vi "Drive Distance Encoder.vi"(0 "Distance (in)":dbl=108.0, 1 "Gyro setpoint":dbl format="%.2f", 5 "Speed":dbl=0.8, 7 "Gyro gains":T1={"proportional gain (Kc)"=-0.08, "integral time (Ti, min)"=0.0, "derivative time (Td, min)"=0.0} {"derivative time (Td, min)" format="%.3f"; "integral time (Ti, min)" format="%.3f"; "proportional gain (Kc)" format="%.3f"}, 9 "Auto Notifiers In":T2, 11 "error in":errorcluster, 12 "Gyro Sync?":bool=TRUE) -> (10 "Auto Notifiers Out":T2, 15 "error out":errorcluster)   [LabVIEW 2014]
doc: "This VI will drive the specified distance at a specified motor output, it will not finish execution until it has reached its destination. The Gyro sync option (True by default) will sync the rotation to the read passed into the vi. Note this is a distance not a displacement (give us a positive)"
uses:
  Auto Notifiers.ctl
  Main/Arms/Arm clapper state.ctl
  Main/Arms/Arm State.ctl
  Utilities/Refname.ctl
  Utilities/Sensor Refname.ctl
  Utilities/RefnameToString.vi
  <vilib>/Rock Robotics/WPI/RobotDrive/WPI_RobotDriveGetSetRefNum.vi
  Utilities/Sensor Refname to String.vi
  <vilib>/addons/control/pid/pid.llb/PID (DBL).vi
  <vilib>/Rock Robotics/WPI/RobotDrive/WPI_RobotDriveArcadeDrive_Standard(NoSaturation).vi
  <vilib>/addons/control/pid/NI_PID_pid.lvlib
panel:
  in  "Max correction rate":dbl=1.0
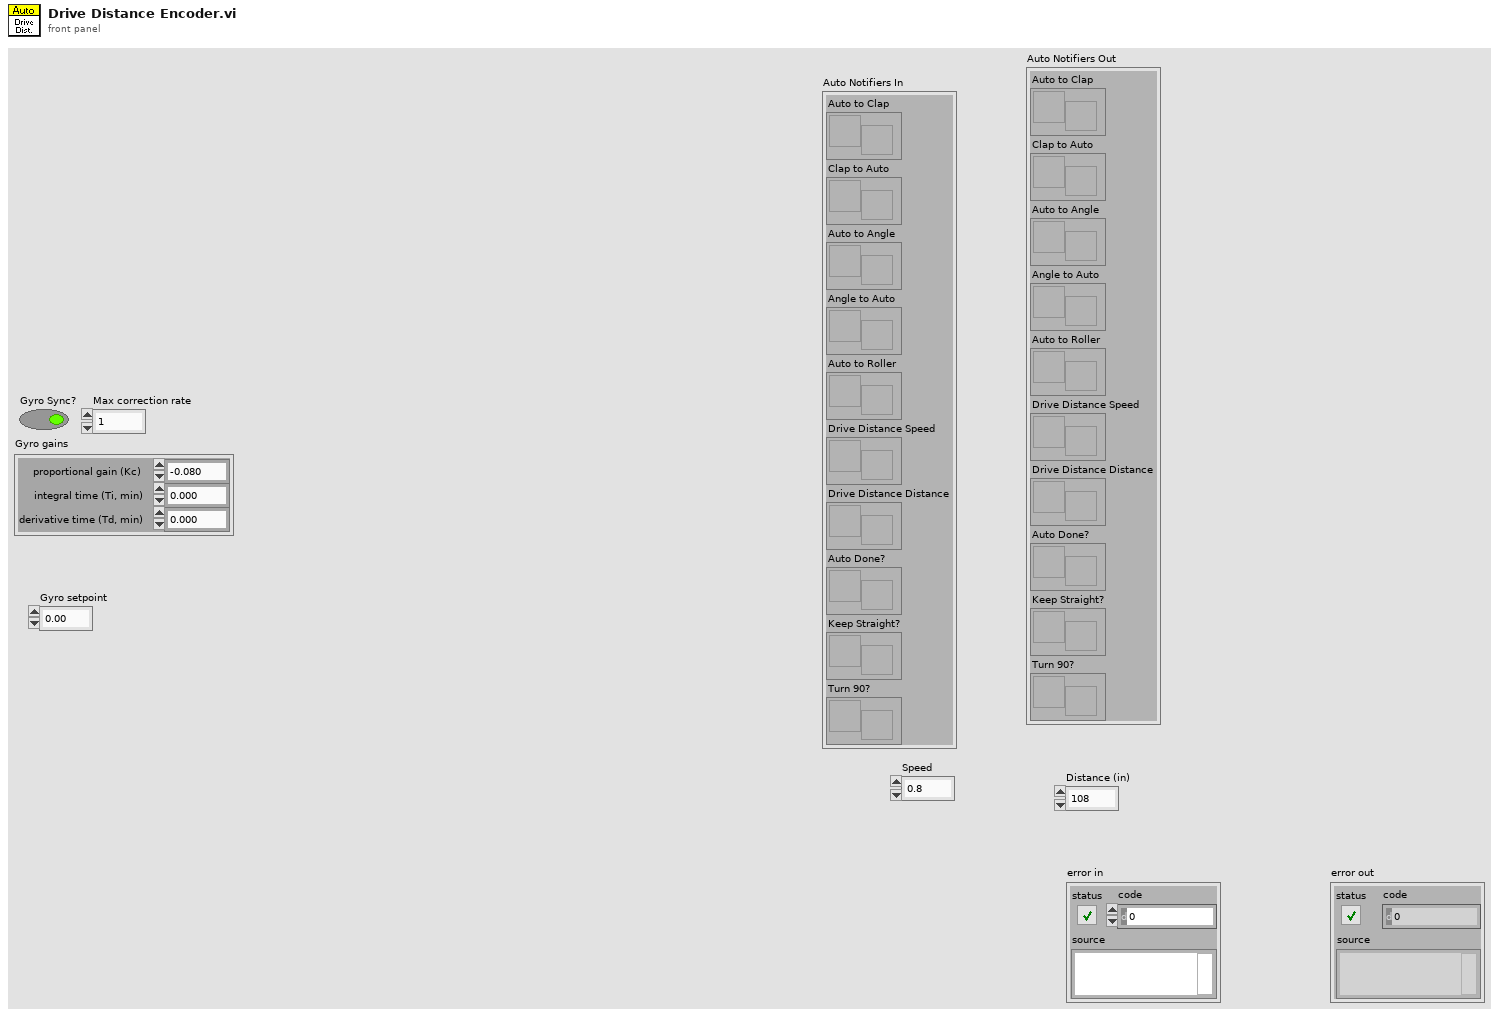
[diagram p1: front panel]
types:
  T1 = cluster{"proportional gain (Kc)":dbl, "integral time (Ti, min)":dbl, "derivative time (Td, min)":dbl}
  T2 = typedef "Auto Notifiers.ctl" = cluster{"Auto to Clap":refnum<notifier>, "Clap to Auto":refnum<notifier>, "Auto to Angle":refnum<notifier>, "Angle to Auto":refnum<notifier>, "Auto to Roller":refnum<notifier>, "Drive Distance Speed":refnum<notifier>, "Drive Distance Distance":refnum<notifier>, "Auto Done?":refnum<notifier>, "Keep Straight?":refnum<notifier>, "Turn 90?":refnum<notifier>}
  T3 = typedef "Refname.ctl" = enum16{"Gamepad 1", "Gamepad 2", "Drive Motors", "Strafe Motor", "Arm Clapper Motor", "Arm Angle", "Arm Belt Left", "Arm Belt Right", "Elevator 1", "Elevator 2", "Wiper"}
  T4 = typedef "WPI_RobotDriveDevRef.ctl" = cluster{"DevStatus":errorcluster, "Motors[]":T5[], "Square Inputs":bool, "Max Output":dbl}
  T5 = typedef "WPI_MotorControlDeviceRef.ctl" = cluster{"DeviceStatus":errorcluster, "Type":T6, "PWM":cluster{"Controller":T7, "PWM Channel":T8, "DeadBand":T9}, "CAN":cluster{"Device Number":u8, "Control Mode":T10, "Semaphore":T11, "Max Vout":dbl, "TalonSRX Control Mode":T12}, "Invert":bool, "TransformRef":T13, "InvTransformRef":T13}
  T6 = typedef "WPI_MotorControlType.ctl" = enum16{"PWM", "CAN", "CANTalonSRX"}
  T7 = typedef "FPGA_TypedefDigitalModule.ctl" = enum16{"Controller 1"}
  T8 = typedef "FPGA_DIOPWMChannel.ctl" = enum8{"PWM 0", "PWM 1", "PWM 2", "PWM 3", "PWM 4", "PWM 5", "PWM 6", "PWM 7", "PWM 8", "PWM 9", "PWM MXP 0", "PWM MXP 1", "PWM MXP 2", "PWM MXP 3", "PWM MXP 4", "PWM MXP 5", "PWM MXP 6", "PWM MXP 7", "PWM MXP 8", "PWM MXP 9", "Invalid"}
  T9 = typedef "WPI_PWMDeadband.ctl" = cluster{"Name":string, "maxPositivePwm":i32, "minPositivePwm":i32, "centerPwm":i32, "maxNegativePwm":i32, "minNegativePwm":i32, "angularRange":u16}
  T10 = typedef "WPI_CANJaguar_ControlMode.ctl" = enum8{"Percent VBus", "Current", "Speed", "Position", "Voltage"}
  T11 = typedef "Semaphore RefNum" = refnum<k1>
  T12 = typedef "WPI_CANTalonSRX_APIControlMode.ctl" = enum8{"Percent VBus", "Speed", "Position", "Slave", "Unchanged / Invalid"}
  T13 = typedef "WPI_PWMTransform_ConPane.ctl" = refnum<vi>
  T14 = typedef "Sensor Refname.ctl" = enum16{"Gyro", "Elevator Top LS", "Elevator Bottom LS", "Claw Outside LS", "Left Drive Encoder", "Right Drive Encoder", "Strafe Encoder", "Elevator Encoder", "Ultrasonic Forward", "Ultrasonic Back", "Arm Angle POT", "Arm Clapper POT", "Accelerometer", "Tote LS", "DIP 1", "DIP 2", "DIP 3", "DIP 4"}
  T15 = typedef "WPI_GyroDevRef.ctl" = cluster{"DevStatus":errorcluster, "Analog Module":T16, "Analog Channel":T17, "Offset":dbl, "Gain (VoltsPerDegree/Second)":dbl}
  T16 = typedef "FPGA_TypedefAnalogModule.ctl" = enum16{"Controller 1"}
  T17 = typedef "FPGA_AIChannel.ctl" = enum8{"AI 0", "AI 1", "AI 2", "AI 3", "AI MXP 0", "AI MXP 1", "AI MXP 2", "AI MXP 3", "Invalid"}
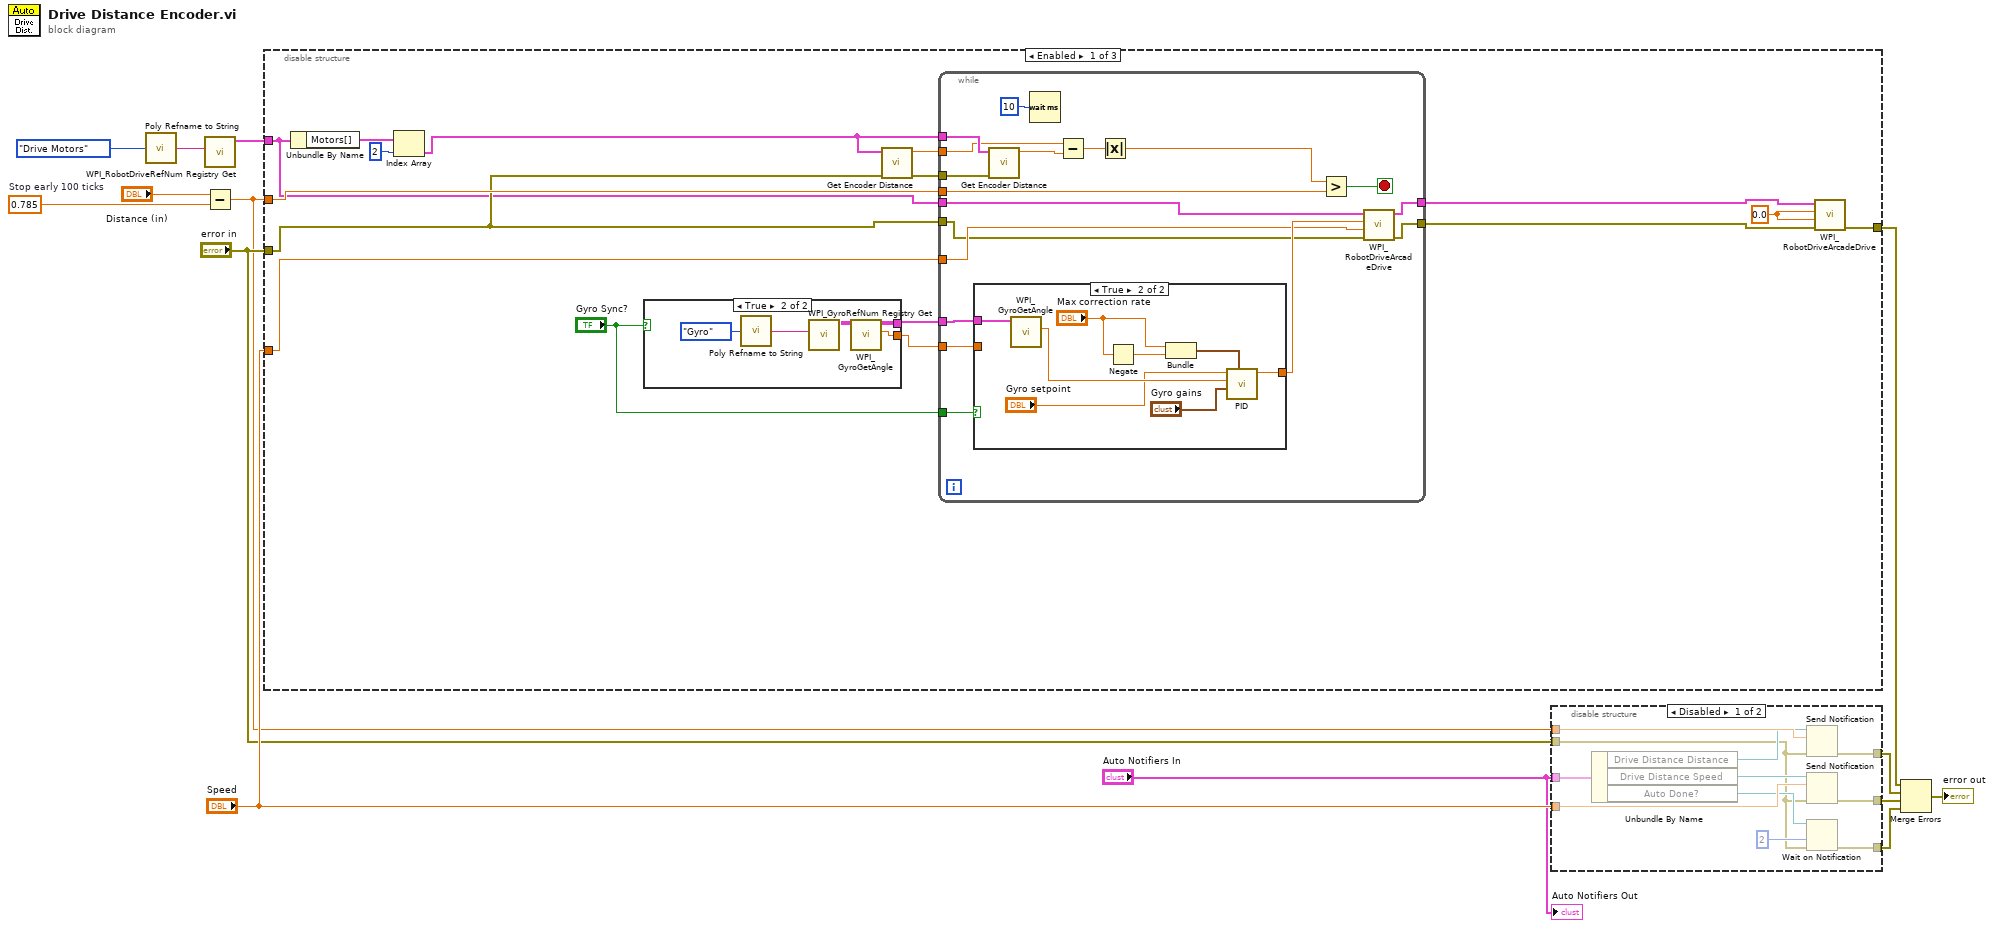
[diagram p0: block diagram]
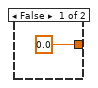
[diagram p4: hidden frame]
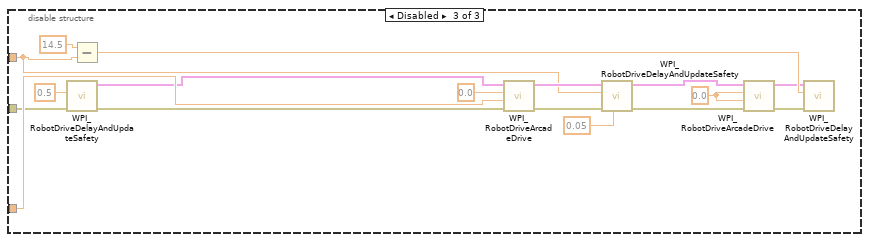
[diagram p6: hidden frame]
diagram:
  w1 = 0.785  # Stop early 100 ticks
  n1 = call-poly "Poly Refname to String.vi"("Enum"=Refname."Drive Motors") -> ("Refname"=w14:string)
  n2 = call <vilib>:"WPI_RobotDriveRefNum Registry Get.vi"("refnum name"=w14) -> ("RobotDriveDevRef"=w12:T4)  [unwired: 9 in, 1 out]
  n3 = Subtract(x="Distance (in)", y=w1) -> (x-y=w2:dbl)
  n4 = disable-structure shown="Enabled" {
    disable-tunnel: w12 -> [w18 _ _]
    disable-tunnel: w2 -> [w23 _ w65]
    disable-tunnel: "error in" -> [w20 _ w72]
    disable-tunnel: [w27 _ _] -> w6
    disable-tunnel: "Speed" -> [w19 _ w75]
    frame Enabled {
      w28 = 0.0 ("X axis value")
      n5 = Unbundle By Name(w18) -> ("Motors[]"=w26:T5[])
      n6 = Index Array(array=w26, index=2) -> (element=w22:T5)
      n7 = case shown="True" "Gyro Sync?" {
        tunnel: [_ w34] -> w16
        tunnel: [_ w33] -> w15
        frame False {
        }
        frame True {
          n8 = call-poly "Poly Refname to String.vi"("Sensor Refnames"=Sensor_Refname."Gyro") -> ("Refname"=w31:string)
          n9 = call <vilib>:"WPI_GyroRefNum Registry Get.vi"("refnum name"=w31) -> ("GyroDevRef"=w35:T15)  [unwired: 9 in, 1 out]
          n10 = call <vilib>:"WPI_GyroGetAngle.vi"("GyroDevRef"=w35) -> ("Angle"=w33:dbl, "GyroDevRef"=w34:T15)  [unwired: 7 in, 2 out]
        }
      }
      n11 = call "Get Encoder Distance.vi"("error in (no error)"=w20, "CAN Talon SRX Ref"=w22) -> ("error out"=w21:errorcluster, "Inches"=w24:dbl)  [unwired: 7 in, 1 out]
      n12 = while {
        tunnel: w24 -> [w52]
        tunnel: w22 -> [w53]
        tunnel: [w39] -> w29
        tunnel: [w38] -> w25
        tunnel: w18 -> [w41]
        tunnel: w23 -> [w49]
        tunnel: w21 -> [w46]
        tunnel: w20 -> [w40]
        tunnel: w19 -> [w43]
        tunnel: "Gyro Sync?" -> [w42]
        tunnel: w16 -> [w37]
        tunnel: w15 -> [w36]
        stop <- w47 stop-if-true
        n13 = case shown="True" w42 {
          tunnel: [0.0 ("X axis value") w62] -> w44
          tunnel: w37 -> [_ w61]
          tunnel: w36 -> [_ _]
          frame False {
          }
          frame True {
            n14 = call <vilib>:"WPI_GyroGetAngle.vi"("GyroDevRef"=w61) -> ("Angle"=w60:dbl)  [unwired: 7 in, 3 out]
            n15 = Negate(x="Max correction rate") -> (-x=w58:dbl)
            n16 = Bundle("Max correction rate"="Max correction rate", w58) -> (w56:cluster{"Max correction rate":dbl, dbl})  [unwired: 1 in]
            n17 = call-poly <vilib>:"PID.vi"("output range"=w56, "PID gains"="Gyro gains", "process variable"=w60, "setpoint"="Gyro setpoint") -> ("output"=w62:dbl)  [unwired: 6 in, 1 out]
          }
        }
        n18 = call "Get Encoder Distance.vi"("error in (no error)"=w46, "CAN Talon SRX Ref"=w53) -> ("Inches"=w51:dbl)  [unwired: 7 in, 2 out]
        n19 = Wait (ms)(milliseconds to wait=u32 10) -> ()  [unwired: 1 out]
        n20 = Subtract(x=w52, y=w51) -> (x-y=w50:dbl)
        n21 = Absolute Value(x=w50) -> (abs(x)=w48:dbl)
        n22 = Greater?(x=w48, y=w49) -> (0:w47:bool)
        n23 = call-poly <vilib>:"WPI_RobotDriveArcadeDrive.vi"("error in (no error)"=w40, "Y axis value"=w43, "X axis value"=w44, "RobotDriveDevRef"=w41) -> ("error out"=w39:errorcluster, "RobotDriveDevRef"=w38:T4)  [unwired: 5 in, 1 out]
      }
      n24 = call-poly <vilib>:"WPI_RobotDriveArcadeDrive.vi"("error in (no error)"=w29, "Y axis value"=w28, "X axis value"=w28, "RobotDriveDevRef"=w25) -> ("error out"=w27:errorcluster)  [unwired: 5 in, 2 out]
    }
    frame Disabled {
    }
    frame Disabled {
      w73 = 0.0 ("X axis value")
      n25 = call <vilib>:"WPI_RobotDriveDelayAndUpdateSafety.vi"("error in (no error)"=w72, "Delay (s)"=0.5) -> ("error out"=w71:errorcluster, "RobotDriveDevRef 2"=w68:T4, "RobotDriveDevRef"=w69:T4)  [unwired: 7 in]
      n26 = Subtract(x=14.5 ("Delay (s)"), y=w65) -> (x-y=w64:dbl)
      n27 = call-poly <vilib>:"WPI_RobotDriveArcadeDrive.vi"("error in (no error)"=w71, "Y axis value"=w75, "X axis value"=0.0, "RobotDriveDevRef"=w68) -> ("error out"=w79:errorcluster, "RobotDriveDevRef"=w78:T4)  [unwired: 5 in, 1 out]
      n28 = call <vilib>:"WPI_RobotDriveDelayAndUpdateSafety.vi"("Feed time (s)"=0.05, "error in (no error)"=w79, "Delay (s)"=w65, "RobotDriveDevRef"=w78) -> ("error out"=w80:errorcluster, "RobotDriveDevRef 2"=w77:T4)  [unwired: 6 in]
      n29 = call-poly <vilib>:"WPI_RobotDriveArcadeDrive.vi"("error in (no error)"=w80, "Y axis value"=w73, "X axis value"=w73, "RobotDriveDevRef"=w77) -> ("error out"=w67:errorcluster, "RobotDriveDevRef"=w63:T4)  [unwired: 5 in, 1 out]
      n30 = call <vilib>:"WPI_RobotDriveDelayAndUpdateSafety.vi"("error in (no error)"=w67, "Delay (s)"=w64, "RobotDriveDevRef"=w63) -> ()  [unwired: 7 in, 2 out]
    }
  }
  n31 = disable-structure shown="Disabled" {
    disable-tunnel: "Speed" -> [w91 _]
    disable-tunnel: w2 -> [w90 _]
    disable-tunnel: "Auto Notifiers In" -> [w89 _]
    disable-tunnel: "error in" -> [w84 _]
    disable-tunnel: [w83 _] -> w5
    disable-tunnel: [w82 _] -> w4
    disable-tunnel: [w81 _] -> w3
    frame Disabled {
      n32 = Unbundle By Name(w89) -> ("Drive Distance Distance"=w88:refnum<notifier>, "Drive Distance Speed"=w87:refnum<notifier>, "Auto Done?"=w86:refnum<notifier>)
      n33 = Send Notification(notification=w90, notifier=w88, error in (no error)=w84) -> (error out=w83:errorcluster)  [unwired: 1 out]
      n34 = Send Notification(notification=w91, notifier=w87, error in (no error)=w84) -> (error out=w82:errorcluster)  [unwired: 1 out]
      n35 = Wait on Notification(notifier=w86, timeout in ms (-1)=2, error in (no error)=w84) -> (error out=w81:errorcluster)  [unwired: 1 in, 3 out]
    }
    frame Enabled {
    }
  }
  n36 = Merge Errors(w6, w5, w4, w3) -> (→"error out":errorcluster)
  "Auto Notifiers Out" <- "Auto Notifiers In"
